vi "spec_protect_detector.vi"(8 "error in (no error)":errorcluster, 9 "protect?":bool, 10 "Detector Name":string, 11 "Qtegra in":refnum<class "Qtegra.lvclass">) -> (0 "error out":errorcluster, 2 "value out":string, 3 "Qtegra out":refnum<class "Qtegra.lvclass">)   [LabVIEW 2017, in "Qtegra.lvclass"]
doc: "Protects/unprotects the detector of the instrument"
uses:
  Qtegra.lvclass
  \\Mac\Home/my data/University/Lamont/Software/LabView/MSControlSuite_Code/MSControl/Classes/Instrument/instrument.lvclass
  global variables.vi
  instrument.lvclass
  StatusLog/StatusLog.lvclass
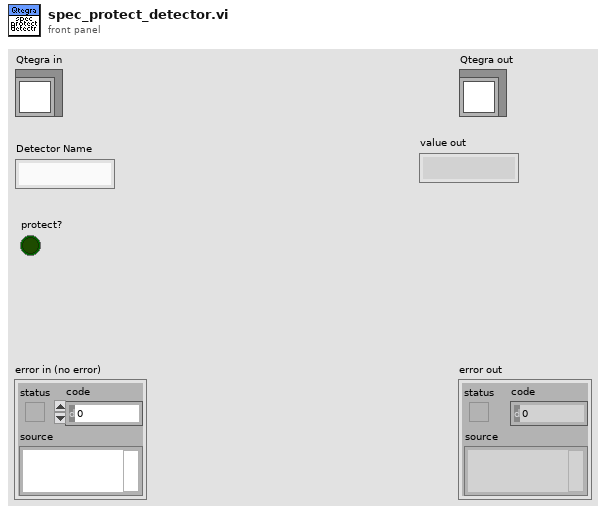
[diagram p1: front panel]
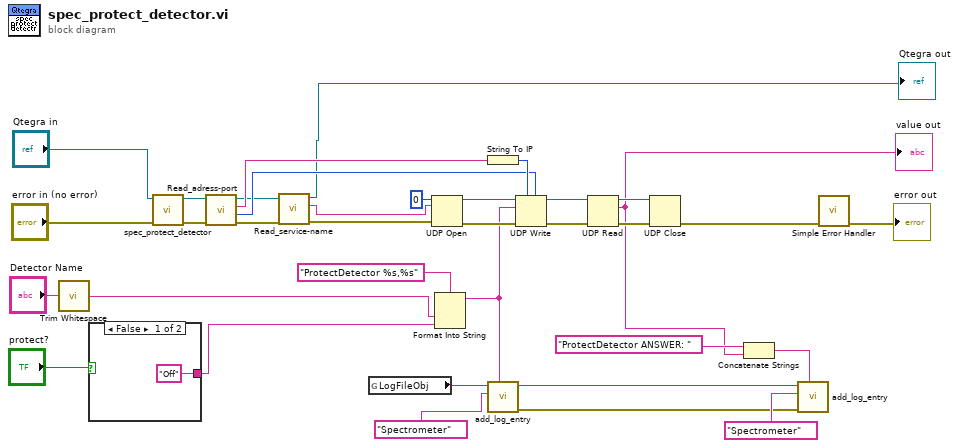
[diagram p0: block diagram]
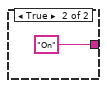
[diagram p2: hidden frame]
diagram:
  n1 = call <vilib>:"Trim Whitespace.vi"("string"="Detector Name") -> ("trimmed string"=w4:string)  [unwired: 1 in]
  n2 = case shown="False" "protect?" {
    tunnel: ["Off" "On"] -> w2
    frame False {
    }
    frame True {
    }
  }
  n3 = call-parent "spec_protect_detector.vi"("error in (no error)"="error in (no error)", "instrument in"="Qtegra in") -> ("error out"=w8:errorcluster, "instrument out"=w9:refnum<class "Qtegra.lvclass">)  [unwired: 7 in, 1 out]
  n4 = call "Read_adress-port.vi"("error in (no error)"=w8, "instrument in"=w9) -> ("error out"=w25:errorcluster, "port number"=w26:i32, "adress"=w33:string, "instrument out"=w24:refnum<class "Qtegra.lvclass">)  [unwired: 6 in]
  n5 = call-dynamic "Read_service-name.vi"("error in (no error)"=w25, "instrument in"=w24) -> ("error out"=w23:errorcluster, "service name"=w22:string, "instrument out"=→"Qtegra out":refnum<class "Qtegra.lvclass">)  [unwired: 7 in]
  n6 = global read "global variables.vi" "LogFileObj"() -> (w15:refnum<class "StatusLog.lvclass">)
  n7 = UDP Open(8:w23, 10:w22, 11:u16 0 ("port")) -> (port=w29:refnum<k16>, 0:w30:errorcluster)  [unwired: 2 in, 1 out]
  n8 = Format Into String(format string="ProtectDetector %s,%s", w4, w2) -> (resulting string=w17:string)  [unwired: 2 in, 1 out]
  n9 = String To IP(1:w33) -> (0:w32:u32)
  n10 = call-dynamic "add_log_entry.vi"("new entry"=w17, "log identifiers"="Spectrometer", "StatusLog in"=w15) -> ("error out"=w10:errorcluster, "StatusLog out"=w14:refnum<class "StatusLog.lvclass">)  [unwired: 5 in]
  n11 = UDP Write(address=w32, port or service name=w26, connection ID=w29, data in=w17, 8:w30) -> (error out=w27:errorcluster, 3:w28:refnum<k16>)  [unwired: 1 in]
  n12 = UDP Read(connection ID=w28, 8:w27) -> (data out=w12:string, error out=w20:errorcluster, 3:w19:refnum<k16>)  [unwired: 2 in, 2 out]
  "value out" <- w12
  n13 = UDP Close(connection ID=w19, 8:w20) -> (error out=w1:errorcluster)  [unwired: 1 out]
  n14 = Concatenate Strings("ProtectDetector ANSWER: ", w12) -> (w11:string)
  n15 = call-dynamic "add_log_entry.vi"("new entry"=w11, "error in (no error)"=w10, "log identifiers"="Spectrometer", "StatusLog in"=w14) -> ()  [unwired: 4 in, 2 out]
  n16 = call <vilib>:"Simple Error Handler.vi"("error in (no error)"=w1) -> ("error out"=→"error out":errorcluster)  [unwired: 4 in, 4 out]
